vi "parse_FeedbackGain.vi"(8 "error in":errorcluster, 11 "msg in":string) -> (0 "error out":errorcluster, 1 "Header":T1, 2 "K":T2, 3 "msg out":string)   [LabVIEW 2018]
uses:
  <vilib>/Analysis/Matrix/Datatypes/RealMatrix.ctl
  <userlib>/ROS for LabVIEW Software/ROS/MessageParsing/std_msgs/subs/parse_float64_array.vi
  <vilib>/Analysis/Matrix/Numeric/Conversions/Array To Matrix - RA2.vi
  <vilib>/Analysis/Matrix/NI_Matrix.lvlib
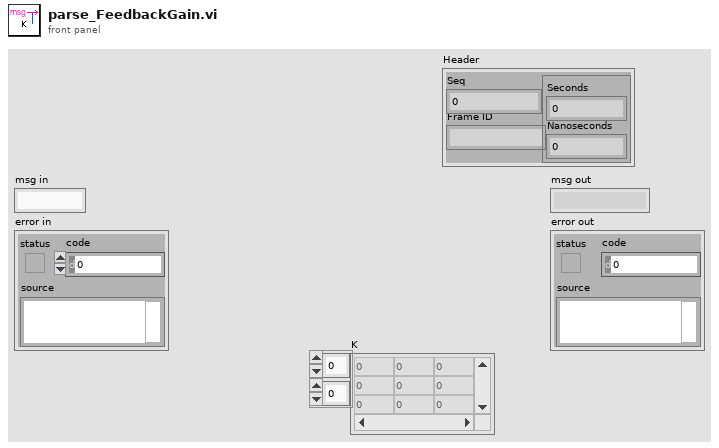
[diagram p1: front panel]
types:
  T1 = cluster{"Seq":u32, "Frame ID":string, "Timestamp":cluster{"Seconds":i32, "Nanoseconds":i32}}
  T2 = typedef "NI_Matrix.lvlib/RealMatrix.ctl" = dbl[][]
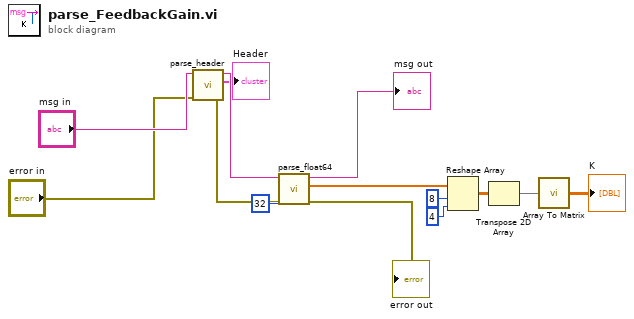
[diagram p0: block diagram]
diagram:
  n1 = call <userlib>:"parse_header.vi"("error in"="error in", "msg in"="msg in") -> ("error out"=w7:errorcluster, "Header"=→"Header":T1, "msg out"=w10:string)  [unwired: 3 in]
  n2 = call-poly <userlib>:"parse_float64.vi"("error in"=w7, "Array Size"=32, "msg in"=w10) -> ("error out"=→"error out":errorcluster, "number"=w6:dbl[], "msg out"=→"msg out":string)  [unwired: 2 in]
  n3 = Reshape Array(w6, 8 ("dimension size"), 4 ("dimension size")) -> (w2:dbl[][])
  n4 = Transpose 2D Array(2D array=w2) -> (transposed array=w1:dbl[][])
  n5 = call-poly <vilib>:"Array To Matrix.vi"("Real 2D Array"=w1) -> ("Real Matrix"=→"K":T2)
